vi "Test Queues.vi"() -> ()   [LabVIEW 2019]
panel:
  in  "stop":bool
  out "dequeue":string
  in  "enqueue":string
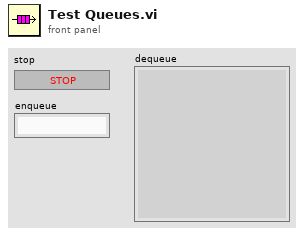
[diagram p1: front panel]
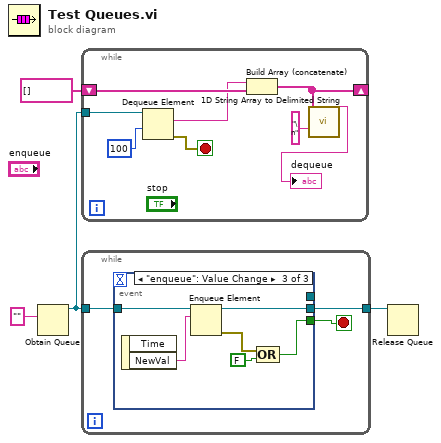
[diagram p0: block diagram]
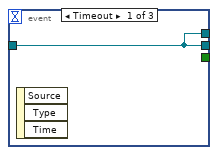
[diagram p2: hidden frame]
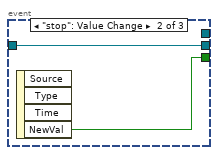
[diagram p3: hidden frame]
diagram:
  n1 = Obtain Queue(element data type="") -> (queue out=w3:refnum<queue>)  [unwired: 4 in, 2 out]
  n2 = while {
    tunnel: w3 -> [w12]
    shift-right: [w7] -> _
    shift-left: string[] [] -> [w10]
    stop <- w11 stop-if-true
    n3 = Dequeue Element(queue=w12, timeout in ms (-1)=100) -> (element=w5:string, error out=w11:errorcluster)  [unwired: 1 in, 2 out]
    n4 = Build Array (concatenate)(w5, w10) -> (w7:string[])
    n5 = call <vilib>:"1D String Array to Delimited String.vi"("delimiter"="\n", "string array"=w7) -> ("delimited string"=→"dequeue":string)  [unwired: 9 in]
  }
  n6 = while {
    tunnel: w3 -> [w15]
    tunnel: [w13] -> w2
    stop <- w14 stop-if-true
    n7 = event shown="[2] \"enqueue\": Value Change" {
      selector: _ -> [_ _ _]
      dyn-events: _ -> [_ _ _]
      timeout: _ -> [_ _ _]
      tunnel: w15 -> [w16 w17 w24]
      tunnel: [w16 _ _] -> _
      tunnel: [_ w18 w20] -> w14
      tunnel: [w16 w17 w19] -> w13
      event Timeout {
        n8 = event-data() -> ()  [unwired: 1 in, 3 out]
      }
      event "stop": Value Change {
        n9 = event-data() -> ("NewVal"=w18:bool)  [unwired: 1 in, 3 out]
      }
      event "enqueue": Value Change {
        n10 = event-data() -> ("NewVal"=w23:string)  [unwired: 1 in, 1 out]
        n11 = Enqueue Element(queue=w24, element=w23) -> (queue out=w19:refnum<queue>, error out=w21:errorcluster)  [unwired: 2 in, 1 out]
        n12 = Compound Arithmetic op=OR(w21, FALSE) -> (w20:bool)
      }
    }
  }
  n13 = Release Queue(queue=w2) -> ()  [unwired: 2 in, 3 out]
